vi "gentec-M-Link.Set Trigger Source.vi"(0 "VISA resource In":refnum<visa-resource-name>, 2 "Trigger Source":T1 items=["Internal", "External"], 5 "error in (no error)":errorcluster) -> (14 "VISA resource Out":refnum<visa-resource-name>, 19 "error out":errorcluster)   [LabVIEW 2014, in "gentec-M-Link - Driver.lvlib"]
doc: "Data to write: src0 or src1\n\nSets the trigger source for energy or radiometric measurement. \n\nsrc0: Trigger source is internal\nsrc1: Trigger source is external"
uses:
  gentec-M-Link - Driver.lvlib
  Type Defs/gentec-M-Link.Trigger Source.ctl
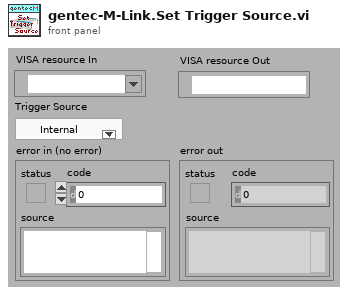
[diagram p1: front panel]
types:
  T1 = typedef "gentec-M-Link - Driver.lvlib/gentec-M-Link.Trigger Source.ctl" = u16
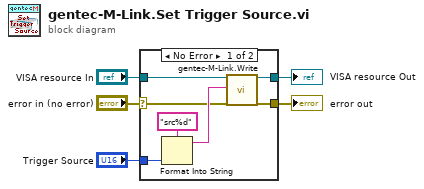
[diagram p0: block diagram]
diagram:
  n1 = case shown="No Error" "error in (no error)" {
    selector: "error in (no error)" -> [w10 w14]
    tunnel: [w6 w14] -> w4
    tunnel: "VISA resource In" -> [w9 w13]
    tunnel: [w7 w13] -> w2
    tunnel: "Trigger Source" -> [w8 _]
    frame No Error {
      n2 = Format Into String(format string="src%d", w8) -> (resulting string=w11:string)  [unwired: 2 in, 1 out]
      n3 = call "gentec-M-Link.Write.vi"("VISA resource (In)"=w9, "Data To Write"=w11, "error in (no error)"=w10) -> ("VISA resource (Out)"=w7:refnum<visa-resource-name>, "error out"=w6:errorcluster)  [unwired: 14 in, 1 out]
    }
    frame Error {
    }
  }
  "error out" <- w4
  "VISA resource Out" <- w2
